vi "Quit Actors.vi"(8 "error in (no error)":errorcluster, 10 "Actor":enum16{"Mixer", "Screw", "Solenoid", "All"}(ring), 11 "Feeder Actor.lvlib:Feeder.lvclass":refnum<class "Feeder.lvclass">) -> (0 "error out":errorcluster, 3 "Feeder Actor.lvlib:Feeder.lvclass 2":refnum<class "Feeder.lvclass">)   [LabVIEW 2018, in "Feeder Actor.lvlib" / "Feeder.lvclass"]
uses:
  Feeder.lvclass
  Feeder.lvclass/Feeder.ctl
  <vilib>/ActorFramework/Message Enqueuer/Message Enqueuer.lvclass/Message Enqueuer.ctl
  <vilib>/ActorFramework/Message Enqueuer/Enqueue.vi
  <vilib>/ActorFramework/Stop Msg/Stop Msg.lvclass
  C:/Program Files/National Instruments/LabVIEW 2018/vi.lib/ActorFramework/Message/Message.lvclass
  <vilib>/ActorFramework/Message Priority Queue/Priority Enqueue.vi
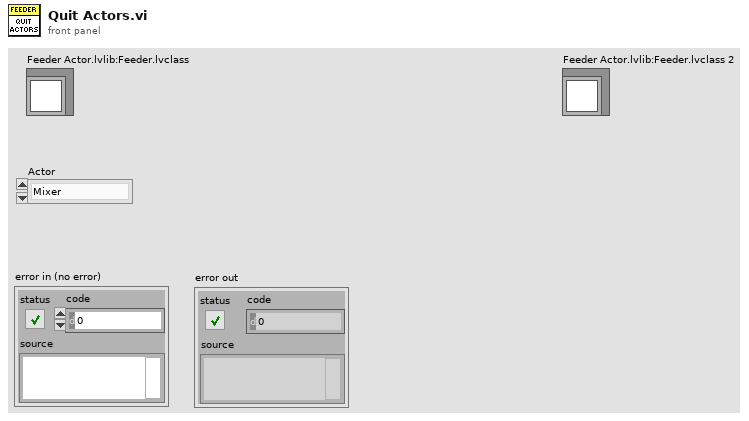
[diagram p1: front panel]
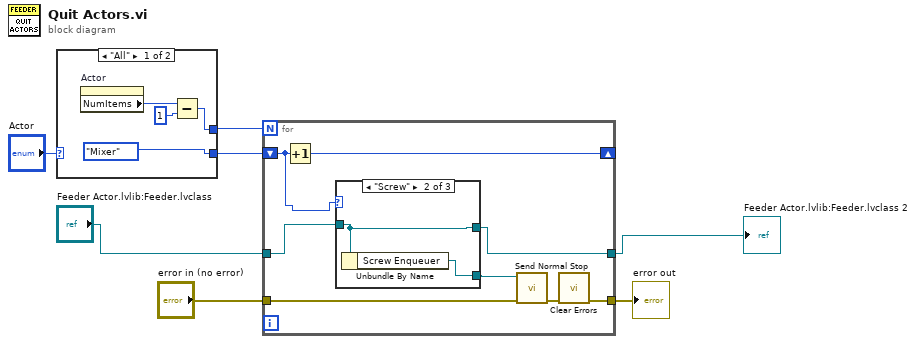
[diagram p0: block diagram]
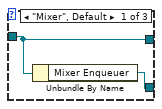
[diagram p2: hidden frame]
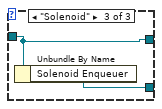
[diagram p3: hidden frame]
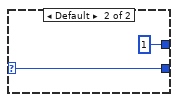
[diagram p4: hidden frame]
diagram:
  n1 = case shown="\"All\"" "Actor" {
    selector: "Actor" -> [_ w12]
    tunnel: [w11 1] -> w5
    tunnel: [enum16{"Mixer", "Screw", "Solenoid", "All"}."Mixer" ("Actor 2") w12] -> w6
    frame "All" {
      n2 = property on="Actor" class="Enum (strict)"() -> ("NumItems"=w10:u32)  [unwired: 2 in, 2 out]
      n3 = Subtract(x=w10, y=u32 1) -> (x-y=w11:u32)
    }
    frame Default {
    }
  }
  n4 = for {
    N: w5 -> [_]
    shift-right: [w21] -> _
    shift-left: w6 -> [w17]
    tunnel: "error in (no error)" -> [w20]
    tunnel: [w18] -> w3
    tunnel: "Feeder Actor.lvlib:Feeder.lvclass" -> [w16]
    tunnel: [w14] -> w1
    n5 = Increment(x=w17) -> (x+1=w21:enum16{"Mixer", "Screw", "Solenoid", "All"})
    n6 = case shown="\"Screw\"" w17 {
      tunnel: w16 -> [w22 w24 w26]
      tunnel: [w23 w25 w27] -> w15
      tunnel: [w22 w24 w26] -> w14
      frame "Mixer", Default {
        n7 = Unbundle By Name(w22) -> ("Mixer Enqueuer"=w23:refnum<class "Message Enqueuer.lvclass">)
      }
      frame "Screw" {
        n8 = Unbundle By Name(w24) -> ("Screw Enqueuer"=w25:refnum<class "Message Enqueuer.lvclass">)
      }
      frame "Solenoid" {
        n9 = Unbundle By Name(w26) -> ("Solenoid Enqueuer"=w27:refnum<class "Message Enqueuer.lvclass">)
      }
    }
    n10 = call <vilib>:"Send Normal Stop.vi"("error in (no error)"=w20, "Message Enqueuer"=w15) -> ("error out"=w19:errorcluster)  [unwired: 9 in]
    n11 = call <vilib>:"Clear Errors.vi"("error in (no error)"=w19) -> ("error out"=w18:errorcluster)  [unwired: 5 in, 1 out]
  }
  "error out" <- w3
  "Feeder Actor.lvlib:Feeder.lvclass 2" <- w1
